vi "Delay.vi"(8 "error in (no error)":errorcluster, 11 "Limit":string) -> (0 "error out":errorcluster, 2 "TestResult":bool, 3 "TestData":string)   [LabVIEW 2013]
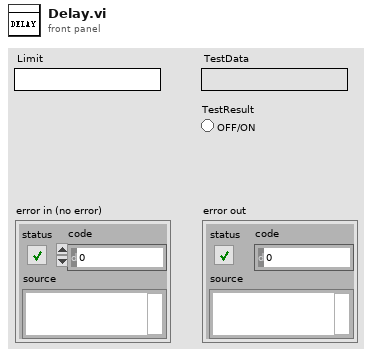
[diagram p1: front panel]
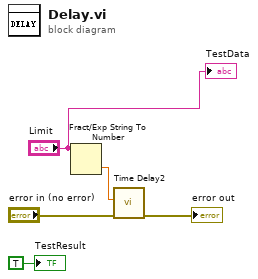
[diagram p0: block diagram]
diagram:
  n1 = Fract/Exp String To Number(string="Limit") -> (number=w2:dbl)  [unwired: 3 in, 1 out]
  n2 = call "Time Delay2"("error in (no error)"="error in (no error)", "Delay Time (s)"=w2) -> ("error out"=→"error out":errorcluster)  [unwired: 9 in]
  "TestData" <- "Limit"
  "TestResult" <- TRUE ("TestResult")
